vi "2023_day14 (SubVI Move Rocks).vi"(1 "Roll Direction":enum16{"north", "west", "south", "east"}(ring), 2 "Map In":string[][](array[string])) -> (7 "Map Out":string[][](array[string]))   [LabVIEW 2021]
uses:
  <userlib>/_OpenG.lib/array/array.llb/Reverse 2D Array (String)__ogtk.vi
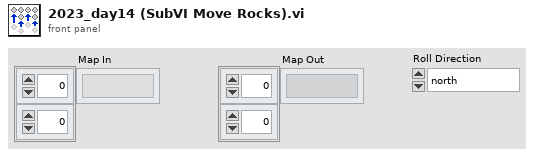
[diagram p1: front panel]
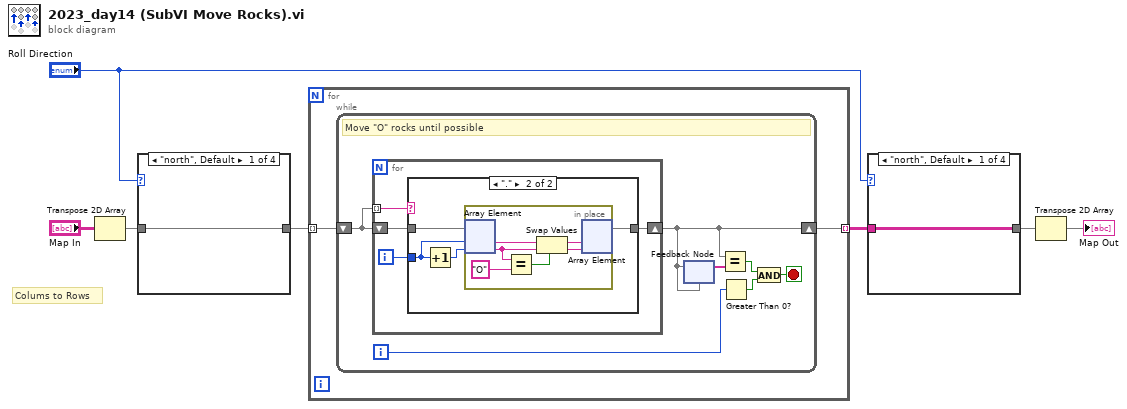
[diagram p0: block diagram]
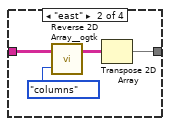
[diagram p2: hidden frame]
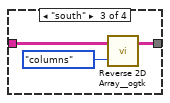
[diagram p3: hidden frame]
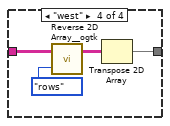
[diagram p4: hidden frame]
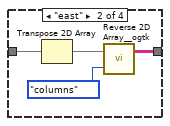
[diagram p5: hidden frame]
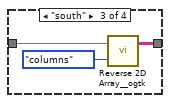
[diagram p6: hidden frame]
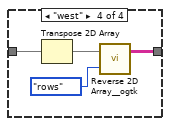
[diagram p7: hidden frame]
diagram:
  # "Colums to Rows"
  n1 = Transpose 2D Array(2D array="Map In") -> (transposed array=w5:string[][])
  n2 = case shown="\"north\", Default" "Roll Direction" {
    tunnel: [w8 w9 w13 w16] -> w4
    tunnel: w5 -> [w8 w12 w14 w19]
    frame "north", Default {
    }
    frame "east" {
      n3 = Transpose 2D Array(2D array=w12) -> (transposed array=w10:string[][])
      n4 = call-poly <userlib>:"Reverse 2D Array__ogtk.vi"("by rows or columns (rows)"=enum16{"rows", "columns"}."columns", "Array"=w10) -> ("Reversed Array"=w9:string[][])  [unwired: 1 in]
    }
    frame "south" {
      n5 = call-poly <userlib>:"Reverse 2D Array__ogtk.vi"("by rows or columns (rows)"=enum16{"rows", "columns"}."columns", "Array"=w14) -> ("Reversed Array"=w13:string[][])  [unwired: 1 in]
    }
    frame "west" {
      n6 = Transpose 2D Array(2D array=w19) -> (transposed array=w17:string[][])
      n7 = call-poly <userlib>:"Reverse 2D Array__ogtk.vi"("by rows or columns (rows)"=enum16{"rows", "columns"}."rows", "Array"=w17) -> ("Reversed Array"=w16:string[][])  [unwired: 1 in]
    }
  }
  n8 = for {
    tunnel: w4 -> [w21] mode=indexing
    tunnel: [w20] -> w3 mode=indexing
    n9 = while {
      shift-right: [w26] -> w20
      shift-left: w21 -> [w28]
      i -> [w25]
      stop <- w22 stop-if-true
      # "Move \"O\" rocks until possible"
      n10 = for {
        tunnel: w28 -> [w32] mode=indexing
        shift-right: [w29] -> w26
        shift-left: w28 -> [w30]
        i -> [w31]
        n11 = case shown="\".\"" w32 {
          tunnel: [w33 w35] -> w29
          tunnel: w31 -> [_ w36]
          tunnel: w30 -> [w33 w37]
          frame Default {
          }
          frame "." {
            n12 = Increment(x=w36) -> (x+1=w34:i32)
            n13 = in-place {
              n14 = in-place-array #1(w37, w36, w34) -> (w41:string, w40:string)
              n15 = Equal?(x=w40, y="O") -> (x = y?=w42:bool)
              n16 = Swap Values(12:w41, 13:w42, 14:w40) -> (1:w38:string, 3:w39:string)
              n17 = in-place-array #1(w38, w39) -> (w35:string[])  [unwired: 2 out]
            }
          }
        }
      }
      n18 = feedback-in #2(w26) -> ()
      n19 = feedback #2(w26) -> (w27:string[])
      n20 = Equal?(x=w26, y=w27) -> (x = y?=w23:bool)
      n21 = Greater Than 0?(x=w25) -> (x > 0?=w24:bool)
      n22 = And(x=w23, y=w24) -> (x .and. y?=w22:bool)
    }
  }
  n23 = case shown="\"north\", Default" "Roll Direction" {
    tunnel: [w44 w45 w49 w54] -> w2
    tunnel: w3 -> [w44 w47 w50 w53]
    frame "north", Default {
    }
    frame "east" {
      n24 = call-poly <userlib>:"Reverse 2D Array__ogtk.vi"("by rows or columns (rows)"=enum16{"rows", "columns"}."columns", "Array"=w47) -> ("Reversed Array"=w46:string[][])  [unwired: 1 in]
      n25 = Transpose 2D Array(2D array=w46) -> (transposed array=w45:string[][])
    }
    frame "south" {
      n26 = call-poly <userlib>:"Reverse 2D Array__ogtk.vi"("by rows or columns (rows)"=enum16{"rows", "columns"}."columns", "Array"=w50) -> ("Reversed Array"=w49:string[][])  [unwired: 1 in]
    }
    frame "west" {
      n27 = call-poly <userlib>:"Reverse 2D Array__ogtk.vi"("by rows or columns (rows)"=enum16{"rows", "columns"}."rows", "Array"=w53) -> ("Reversed Array"=w52:string[][])  [unwired: 1 in]
      n28 = Transpose 2D Array(2D array=w52) -> (transposed array=w54:string[][])
    }
  }
  n29 = Transpose 2D Array(2D array=w2) -> (transposed array=→"Map Out":string[][])
